vi "PSTR Offline Analysis.vi"() -> ()   [LabVIEW 2020]
uses:
  <vilib>/printing/EasyPrintingControls.llb/layout_options.ctl
  <vilib>/printing/EasyPrintingControls.llb/orientation.ctl
  <vilib>/printing/EasyPrintingControls.llb/panel_scaling_for_page.ctl
  <vilib>/printing/EasyPrintingControls.llb/margins.ctl
  <vilib>/printing/EasyPrintingControls.llb/margin_values.ctl
  <vilib>/printing/EasyPrintingControls.llb/measurement_system.ctl
  <vilib>/printing/EasyPrintingControls.llb/printer_options.ctl
  <vilib>/printing/EasyPrintingControls.llb/printing_method.ctl
  <vilib>/printing/EasyPrintingControls.llb/color_or_monochrome.ctl
  <vilib>/printing/EasyPrintingControls.llb/page_header_options.ctl
  <vilib>/printing/EasyPrintingControls.llb/page_headers.ctl
  <vilib>/printing/EasyPrintingControls.llb/page_header_content_options.ctl
  PSTR VIs/Typedefs/PSTR-Data.ctl
  PSTR VIs/Typedefs/PSTR-Model Fit.ctl
  PSTR VIs/Typedefs/PSTR-Fit Parameters.ctl
  Utility VIs/Buttons/KCheckmarkBoolean 2.ctl
  PSTR VIs/Typedefs/PSTR-File Info.ctl
  PSTR VIs/Typedefs/PSTR-Parameters.ctl
  PSTR VIs/Typedefs/PSTR-Stimulus Params.ctl
  Utility VIs/Type Defs/Left-Right ring.ctl
  PSTR VIs/Typedefs/PSTR-FreqSeq Params.ctl
  PSTR VIs/Typedefs/PSTR-LevelSeq Params.ctl
  PSTR VIs/Typedefs/PSTR-SeqParams.ctl
  PSTR VIs/Typedefs/PSTR-Response Params.ctl
  PSTR VIs/Typedefs/PSTR-Hidden Params.ctl
  PSTR VIs/Typedefs/PSTR-Window Shape.ctl
  Typedefs/PSTRA-Analysis State.ctl
  <vilib>/printing/EasyPrintingControls.llb/contents.ctl
  <vilib>/printing/EasyPrinting.llb/Easy Print VI Panel or Documentation (refnum).vi
  <vilib>/Utility/NIReport.llb/NI_ReportGenerationCore.lvlib
panel:
  out "CFTS-PSTR":T1
  in  "Mat Button":bool
  out "progress":dbl(slide) caption="2 kHz" scale=0.0..1.0
  in  "Reanalyze Button":bool
  out "Info":string
  in  "Path":path
  in  "Response":T2={"Grass gain"=10000.0, "Window (ms)"=10000.0, "Window shape"=enum."NONE", "NFFT"=10000}
  in  "Cancel Button":bool
  in  "Tabs":enum32{"Gain", "PSTR"}(tab)
  out "Spectrum":cluster{dbl, "dx":dbl, "Y":dbl[]}[](graph)
  out "vsFreq":cluster{"Array":dbl[], "Array":dbl[]}[](graph)
  in  "Legend":i32(listbox)
  out "Gain":cluster{"Array":dbl[], "Array":dbl[]}[](graph)
  in  "iFreq":u16(ring) items=["2 kHz"]
  out "RespAmp":cluster{"Array":dbl[], "Array":dbl[]}[](graph)
  in  "Show fits":T3
  in  "iFreq 2":u16(ring) items=["2 kHz"]
  in  "Legend 2":i32(listbox)
  in  "Separation (uV)":dbl min=0.0 step=1.0
  out "FitSummary":cluster{"Array":dbl[], "Array":dbl[]}[](graph)
  out "PSTH":cluster{"Array":dbl[], "Array":dbl[]}[](graph)
  out "finished":errorcluster
  out "Result":cluster{"Data":T4, "error":errorcluster}
  in  "layout options":T7={"orientation (unchanged)"=0, "panel scaling for page (unchanged)"=0, "margins"={"override VI margins (false)"=FALSE, "margins (1.00)"={"top"=1.0, "left"=1.0, "right"=1.0, "bottom"=1.0}, "measurement system (default)"=0}, "printer options"={"destination printer name (current)"="", "printing method (unchanged)"=0, "color or monochrome (unchanged)"=0}, "page header options"={"page headers (unchanged)"=0, "page header content options"={"Include VI Name"=TRUE, "Include VI Path"=TRUE, "Include Last Modification Date"=TRUE, "Include Date Printed"=TRUE, "Include Page Number"=TRUE, "Include VI Icon"=TRUE}}} {"page header options"."page headers (unchanged)" items=["Unchanged", "Include page headers", "Do not include page headers"]; "printer options"."color or monochrome (unchanged)" items=["Unchanged", "Color/grayscale", "Monochrome"]; "printer options"."printing method (unchanged)" items=["Unchanged", "Standard", "PostScript", "Bitmap"]; "panel scaling for page (unchanged)" items=["Unchanged", "No Scaling", "Scale front panel to fit"]; "orientation (unchanged)" items=["Unchanged", "portrait", "landscape"]; "margins"."measurement system (default)" items=["Default", "US", "Metric"]; "margins"."margins (1.00)"."right" format="%.2f"; "margins"."margins (1.00)"."bottom" format="%.2f"; "margins"."margins (1.00)"."top" format="%.2f"; "margins"."margins (1.00)"."left" format="%.2f"}
  # "PSTR Analysis"
  # "NF x NL x 2 x Npts"
  # "NF x NL x Npts"
  # "NF x NL"
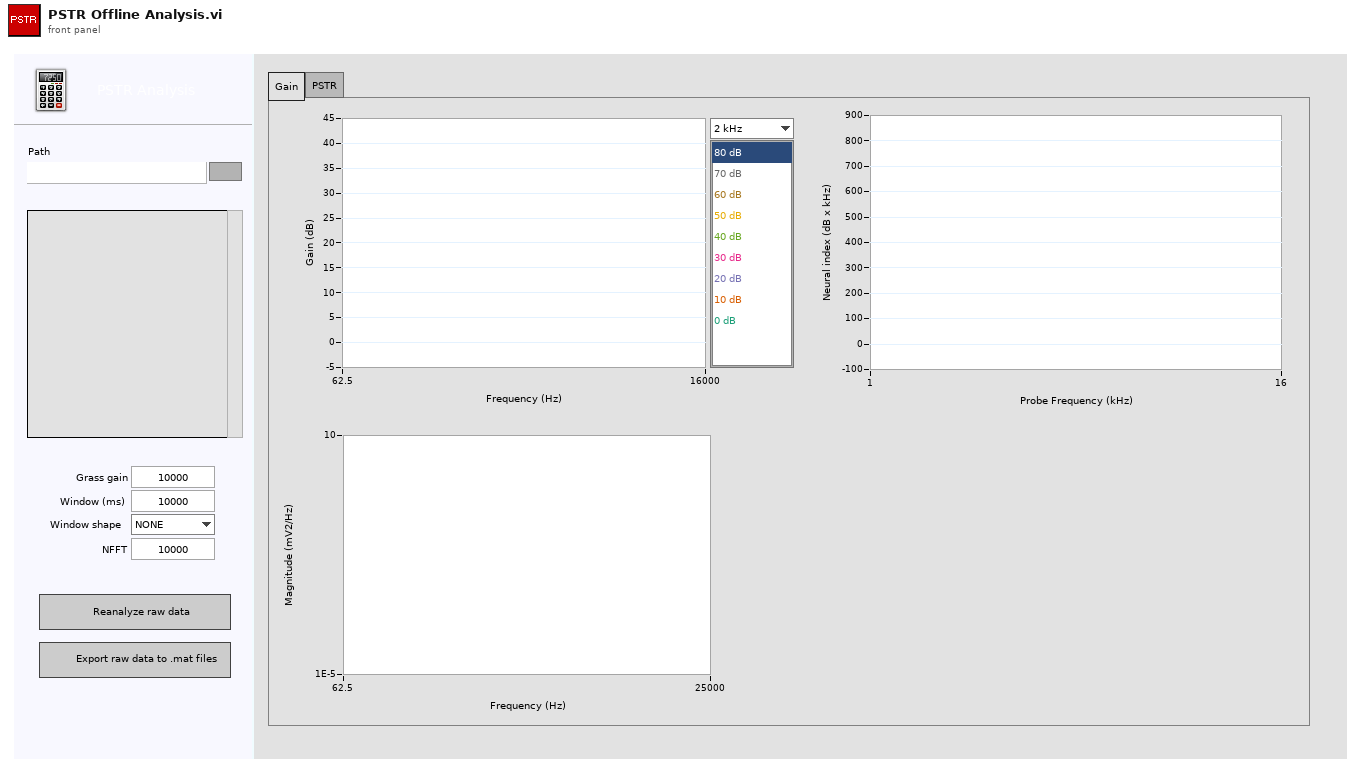
[diagram p1: front panel]
types:
  T1 = typedef "PSTR-File Info.ctl" = cluster{"Date":string, "Filename":string, "Version":i32, "Notes":string}
  T2 = cluster{"Grass gain":dbl, "Window (ms)":dbl, "Window shape":enum16{"NONE", "Hamming"}, "NFFT":i32}
  T3 = typedef "KCheckmarkBoolean 2.ctl" = bool
  T4 = typedef "PSTR-Data.ctl" = cluster{"Freq":dbl[], "Level":dbl[], "order":i32[], "PSD":dbl[][][][], "Gain":dbl[][][], "Index":dbl[][], "iFreq":i32, "df":dbl, "User":string, "ID":i32, "Run":i32, "iLevel":i32, "finished":bool, "resumed":bool, "Spont":dbl[][], "PSTR":dbl[][][], "dt":dbl, "delay":dbl, "durat":dbl, "Fits":T5[][], "Amplitude":dbl[][]}
  T5 = typedef "PSTR-Model Fit.ctl" = cluster{"Parameters":T6, "t":dbl[], "y":dbl[], "R2":dbl}
  T6 = typedef "PSTR-Fit Parameters.ctl" = cluster{"Ar":dbl, "Tr":dbl, "Ast":dbl, "Tst":dbl, "Ass":dbl}
  T7 = typedef "NI_ReportGenerationCore.lvlib/layout_options.ctl" = cluster{"orientation (unchanged)":T8, "panel scaling for page (unchanged)":T9, "margins":T10, "printer options":T13, "page header options":T16}
  T8 = typedef "NI_ReportGenerationCore.lvlib/orientation.ctl" = u16
  T9 = typedef "NI_ReportGenerationCore.lvlib/panel_scaling_for_page.ctl" = u16
  T10 = typedef "NI_ReportGenerationCore.lvlib/margins.ctl" = cluster{"override VI margins (false)":bool, "margins (1.00)":T11, "measurement system (default)":T12}
  T11 = typedef "NI_ReportGenerationCore.lvlib/margin_values.ctl" = cluster{"top":dbl, "left":dbl, "right":dbl, "bottom":dbl}
  T12 = typedef "NI_ReportGenerationCore.lvlib/measurement_system.ctl" = u16
  T13 = typedef "NI_ReportGenerationCore.lvlib/printer_options.ctl" = cluster{"destination printer name (current)":string, "printing method (unchanged)":T14, "color or monochrome (unchanged)":T15}
  T14 = typedef "NI_ReportGenerationCore.lvlib/printing_method.ctl" = u16
  T15 = typedef "NI_ReportGenerationCore.lvlib/color_or_monochrome.ctl" = u16
  T16 = typedef "NI_ReportGenerationCore.lvlib/page_header_options.ctl" = cluster{"page headers (unchanged)":T17, "page header content options":T18}
  T17 = typedef "NI_ReportGenerationCore.lvlib/page_headers.ctl" = u16
  T18 = typedef "NI_ReportGenerationCore.lvlib/page_header_content_options.ctl" = cluster{"Include VI Name":bool, "Include VI Path":bool, "Include Last Modification Date":bool, "Include Date Printed":bool, "Include Page Number":bool, "Include VI Icon":bool}
  T19 = typedef "PSTRA-Analysis State.ctl" = cluster{"Last folder":path, "separation":dbl}
  T20 = typedef "PSTR-Parameters.ctl" = cluster{"Stimulus":T21, "FreqSeq":T23, "LevelSeq":T24, "Seq":T25, "Response":T26, "Hidden":T27, "RejThr":dbl}
  T21 = typedef "PSTR-Stimulus Params.ctl" = cluster{"Ear":T22, "BW (oct)":dbl, "Seed":i32, "Ramp (ms)":dbl, "On time (ms)":dbl, "Off time (ms)":dbl, "Delay (ms)":dbl}
  T22 = typedef "Left-Right ring.ctl" = enum16{"Right", "Left"}
  T23 = typedef "PSTR-FreqSeq Params.ctl" = cluster{"Min (kHz)":dbl, "Max (kHz)":dbl, "Step (oct)":dbl}
  T24 = typedef "PSTR-LevelSeq Params.ctl" = cluster{"Min (dB)":dbl, "Max (dB)":dbl, "Step (dB)":dbl}
  T25 = typedef "PSTR-SeqParams.ctl" = cluster{"Order":enum16{"Sequential", "Random"}, "Averages":i32}
  T26 = typedef "PSTR-Response Params.ctl" = cluster{"Grass gain":dbl, "Window (ms)":dbl}
  T27 = typedef "PSTR-Hidden Params.ctl" = cluster{"Sample rate (Hz)":dbl, "Nfft":i32, "save raw":bool, "sep":dbl, "Window":T28}
  T28 = typedef "PSTR-Window Shape.ctl" = enum16{"NONE", "Hamming"}
  T29 = cluster{enum16{"Reprocess", "Export"}, path, "PSTR Params":T20}
  T30 = typedef "PSTR-SCL Element.ctl" = cluster{"raw file":path, "iFreq":i32, "iLevel":i32, "spont":bool}
  T31 = typedef "PSTR-Runtime Data.ctl" = cluster{"Fs":dbl, "AOpts":i32, "stimChan":T32, "len":i32, "offset1":i32, "iLevel":i32, "AOChan":i32[], "Level":dbl[], "nacc":i32, "nrej":i32, "nacq":i32, "abort":bool, "offset2":i32, "gain":dbl, "Nfft":i32, "Neural":dbl[], "Micro":dbl[], "raw":refnum<file>, "spont":bool, "PSTR":dbl[], "trialLen":i32, "gate":dbl[], "window":u16, "BP":cluster{"reverse":dbl[], "forward":dbl[]}, "Smooth":cluster{"reverse":dbl[], "forward":dbl[]}}
  T32 = typedef "Stimulus Channel (Full).xctl/Full Stimulus Channel Data.ctl" = cluster{"Waveform":T33, "Filter":T50, "Burst":T52, "Level":T53, "Name":string, "Advanced":T55, "SAM":T56}
  T33 = typedef "Waveform XCtl.xctl/Waveform Data.ctl" = cluster{"Type":T34, "Tone":T35, "Pulse Train":T36, "Noise":T39, "File":T40, "FMSweep":T41, "Chirp Train":T42, "Complex Tone":cluster{"Params":T44, "Data":T46}, "Moving Ripple":T47}
  T34 = typedef "Waveform Enum.ctl" = enum16{"OFF", "Tone", "Noise", "Pulse Train", "File", "FM Sweep", "Chirp Train", "Complex Tone", "FM Tone", "Moving Ripple"}
  T35 = typedef "Tone Params.ctl" = cluster{"Frequency (kHz)":dbl, "Last Freq":dbl, "Last Phase":dbl}
  T36 = typedef "Pulse Train Params.ctl" = cluster{"Pulse width (us)":dbl, "Pulse rate (Hz)":dbl, "Gap (ms)":dbl, "Polarity":T37, "PT State":T38, "Asynch":bool}
  T37 = typedef "Pulse Polarity.ctl" = enum16{"POS", "NEG", "POS-NEG", "NEG-POS"}
  T38 = typedef "PT-Continuous State.ctl" = cluster{"Template":dbl[], "Nperiod":i32, "Index":i32, "Pulse Rate (Hz)":dbl, "Phase (cycles)":dbl, "Noff":i32}
  T39 = typedef "Noise Params.ctl" = cluster{"InvFilt":bool, "Noise":dbl[], "CurPt":i32, "Aweight":bool, "Seed":i32, "afile":path}
  T40 = typedef "StimFile-Params.ctl" = cluster{"Filename":path, "Signal":dbl[], "Channel":i32, "stream":bool, "offset":i32, "nreps":i32, "loops":i32, "Randomize":bool, "order":i32[], "Seed":i32, "Tokens":i32}
  T41 = typedef "FM Sweep Params.ctl" = cluster{"Rate (oct/s)":dbl, "Fmin (Hz)":dbl, "Fmax (Hz)":dbl, "Ramp (ms)":dbl, "Linear":bool}
  T42 = typedef "Chirp Train.ctl" = cluster{"Params":T43, "Data":cluster{"WF":dbl[]}}
  T43 = typedef "Chirp Train Params.ctl" = cluster{"Fmin (kHz)":dbl, "Fmax (kHz)":dbl, "Compensate":bool, "Duration (ms)":dbl}
  T44 = typedef "CT-Params.ctl" = cluster{"F0 (Hz)":dbl, "Band":cluster{"Flow (Hz)":dbl, "Fhigh (Hz)":dbl}, "Phase":T45, "Min F0 (Hz)":dbl, "Max F0 (Hz)":dbl, "ContinRandPhase":bool, "Max peak factor":dbl, "Max mod depth":dbl, "MinHarmNum":i32, "MaxHarmNum":i32, "Level Mode":enum16{"per component", "overall rms"}, "% jitter":dbl}
  T45 = typedef "CT-Phase Enum.ctl" = enum16{"Cosine", "Random", "Alternating"}
  T46 = typedef "CT-Runtime Data.ctl" = cluster{"Ncomp":i32, "MinHarm":i32, "Phase":dbl[], "Amplitude":dbl[], "Npts/frame":i32, "Last F0":dbl, "Fmin":dbl, "Fmax":dbl, "Lslope":dbl, "randphase":bool, "overall rms":bool, "fmult":dbl[], "jittered":bool}
  T47 = typedef "Moving Ripple.ctl" = cluster{"Params":T48, "Data":T49}
  T48 = typedef "Moving Ripple.Params.ctl" = cluster{"Fmin":dbl, "Fmax":dbl, "Density":dbl, "Velocity":dbl, "Depth":dbl, "Phase":dbl, "Comp/oct":i32}
  T49 = typedef "Moving Ripple.Data.ctl" = cluster{"Freq":dbl[], "A":dbl[], "phase":dbl[], "Phase":dbl}
  T50 = typedef "Advanced Filter XCtl.xctl/Filter Data.ctl" = cluster{"Type":enum16{"Lowpass", "Highpass", "Bandpass", "Bandstop", "OFF"}, "CF (kHz)":dbl, "BW (kHz)":dbl, "Cascade":bool, "Quadrature":bool, "Scale Factor":dbl, "Stages":cluster{"IIR Filter":cluster{"filter structure":enum32{"IIR 2nd Order", "IIR 4th Order"}, "Reverse Coefficients":dbl[], "Forward Coefficients":dbl[]}, "State":dbl[]}[], "Class":enum16{"Elliptic", "Butterworth"}, "Order":i32, "BWUnits":T51}
  T51 = typedef "Filter-Bandwidth Units.ctl" = enum16{"Linear", "Octaves", "Min-Max"}
  T52 = typedef "Burst Control.xctl/Burst Data.ctl" = cluster{"Active":bool, "Delay (ms)":dbl, "Duration (ms)":dbl, "Ramp (ms)":dbl, "Rate (Hz)":dbl, "Trepeat (ms)":dbl, "Repeat":bool}
  T53 = typedef "Level XCtl.xctl/Level Data.ctl" = cluster{"Level":dbl, "Units":T54, "Max":dbl, "Multiplier":dbl, "Cal File":path, "Cal":cluster{"Freq (Hz)":dbl[], "Mag (dB SPL)":dbl[], "Phase (deg)":dbl[]}}
  T54 = typedef "Level Units.ctl" = enum16{"dB atten", "dB SPL", "dB re 1 Vrms", "dB V/Hz½", "mW", "dB HL", "Volts", "dB mW"}
  T55 = typedef "Advanced Stimulus Options.xctl/Advanced Stimulus Options.ctl" = cluster{"Rep Mask":string, "AltPol":bool, "Var":string, "Expr":string, "Persist":bool}
  T56 = typedef "SAM Params.ctl" = cluster{"Active":bool, "Frequency (Hz)":dbl, "Depth":dbl, "Init Phase (cycles)":dbl, "phase (degrees)":dbl, "Asynch":bool}
  T57 = enum8{"Enabled", "Disabled", "Disabled and Grayed Out"}
  T58 = typedef "NI_ReportGenerationCore.lvlib/contents.ctl" = u16
  T59 = cluster{enum16{"Reprocess", "Export"}, "Path":path, "PSTR Params":T20}
  T60 = cluster{"Grass gain":dbl, "Window (ms)":dbl, "Window":T28, "Nfft":i32}
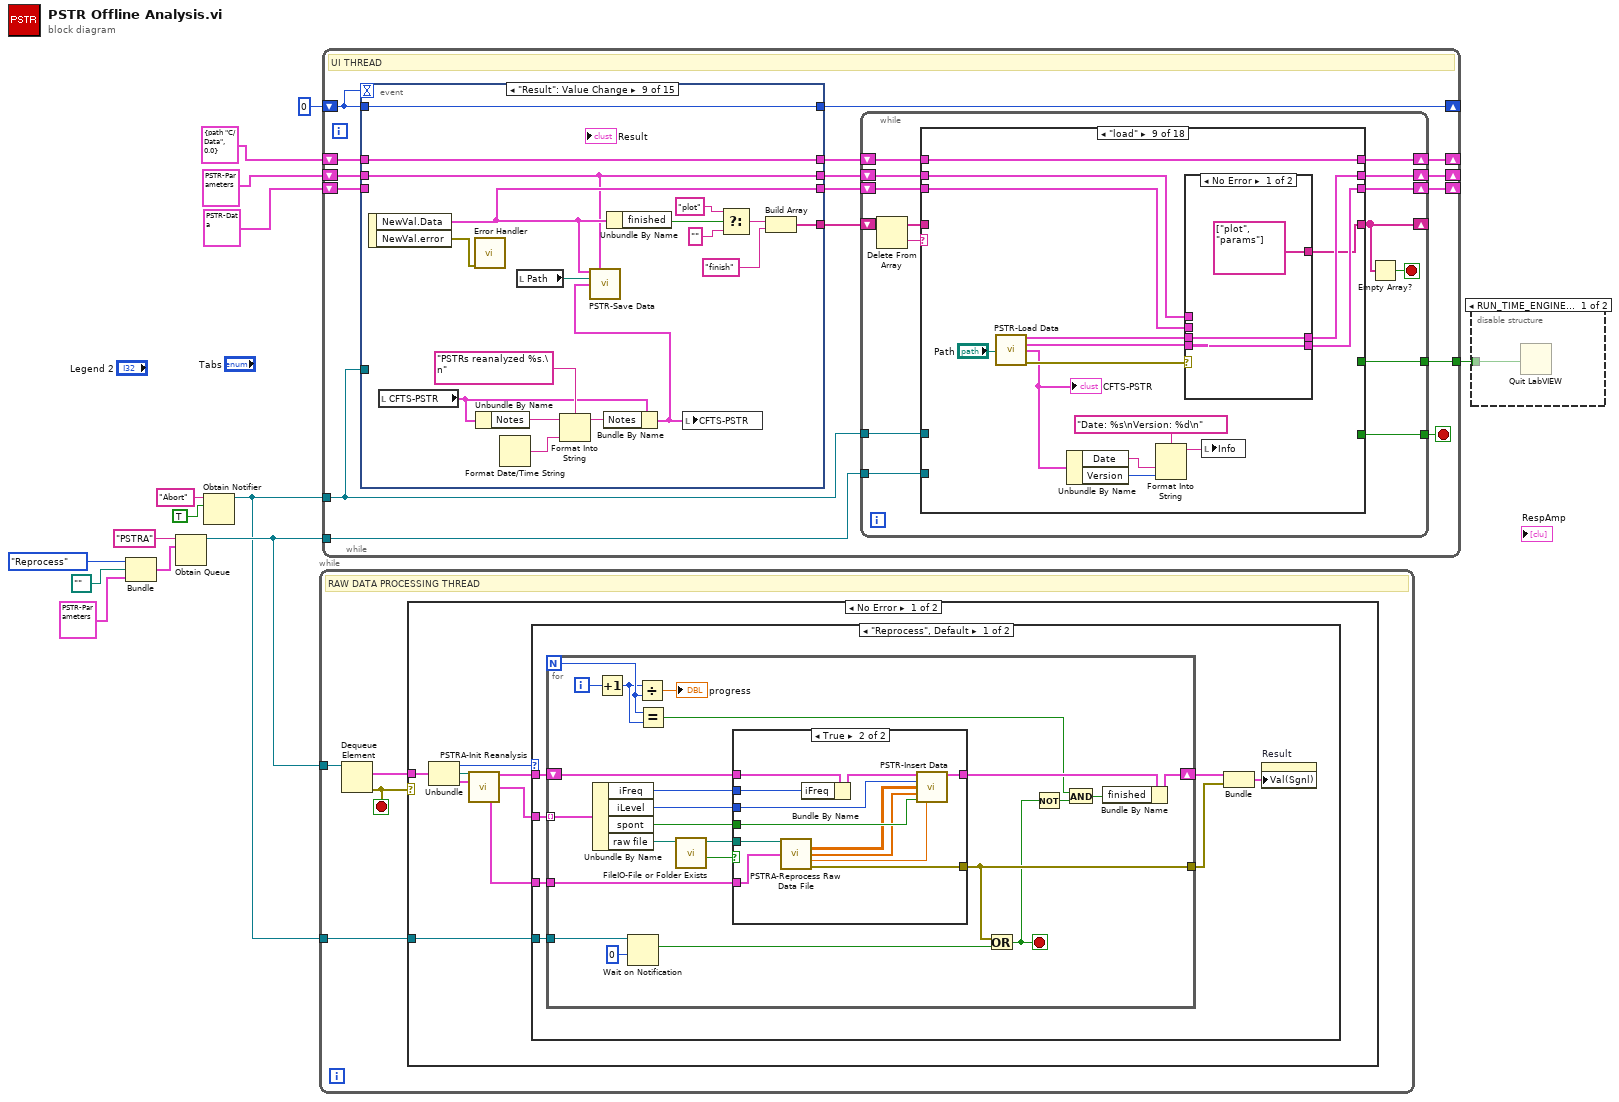
[diagram p0: block diagram]
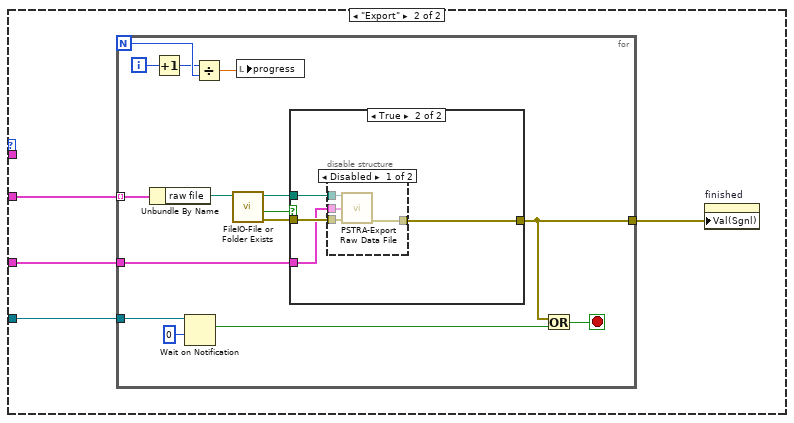
[diagram p4: hidden frame]
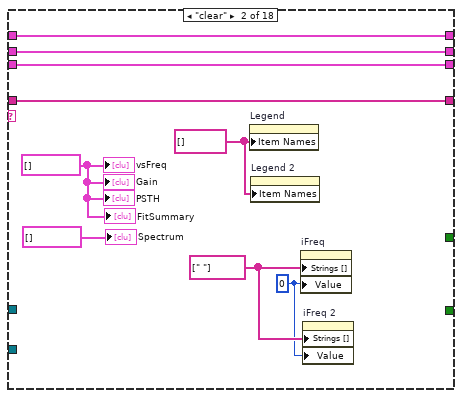
[diagram p9: hidden frame]
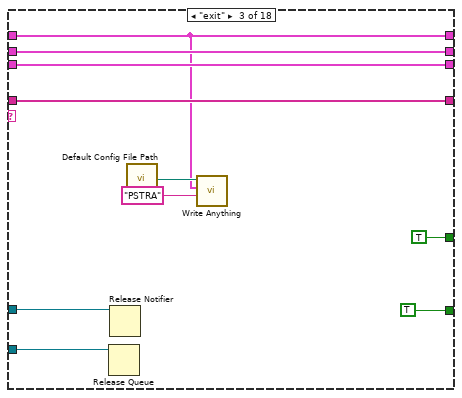
[diagram p10: hidden frame]
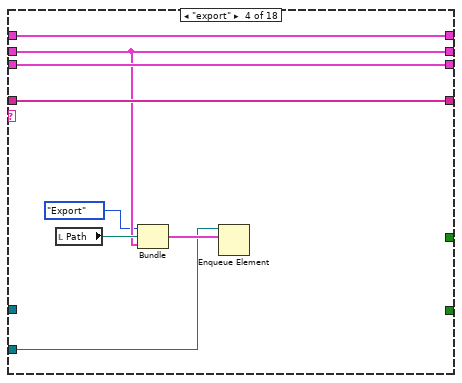
[diagram p11: hidden frame]
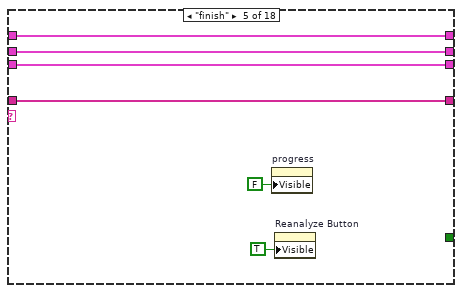
[diagram p12: hidden frame]
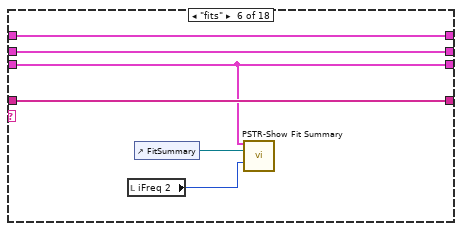
[diagram p13: hidden frame]
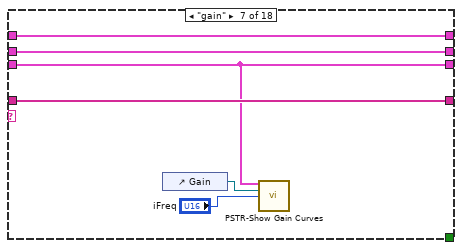
[diagram p14: hidden frame]
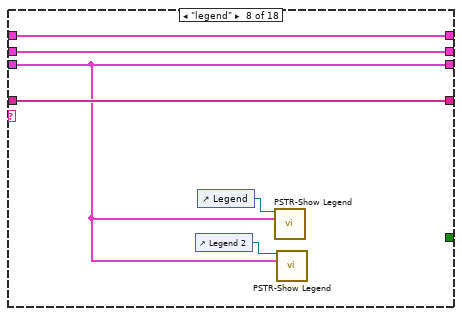
[diagram p15: hidden frame]
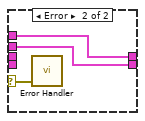
[diagram p16: hidden frame]
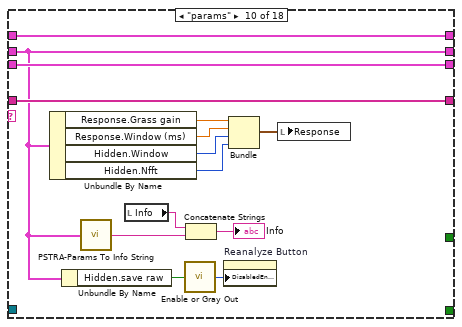
[diagram p17: hidden frame]
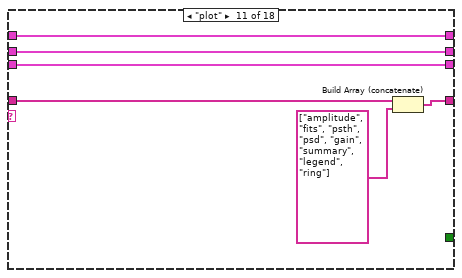
[diagram p18: hidden frame]
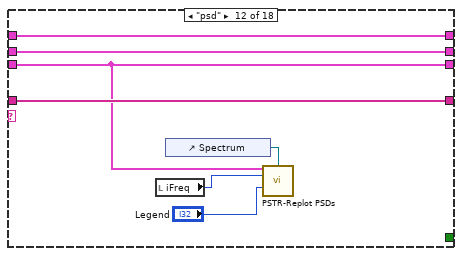
[diagram p19: hidden frame]
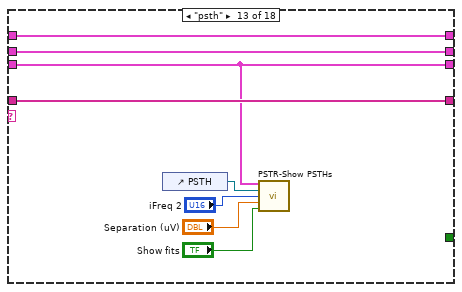
[diagram p20: hidden frame]
diagram:
  n1 = Bundle(enum16{"Reprocess", "Export"}."Reprocess", path "", "PSTR Params"=T20 {"Stimulus"={"Ear"=enum."Right", "BW (oct)"=673.0, "Seed"=6, "Ramp (ms)"=10000.0, "On time (ms)"=10000.0, "Off time (ms)"=10000.0, "Delay (ms)"=10000.0}, "FreqSeq"={"Min (kHz)"=10000.0, "Max (kHz)"=10000.0, "Step (oct)"=10000.0}, "LevelSeq"={"Min (dB)"=10000.0, "Max (dB)"=10000.0, "Step (dB)"=10000.0}, "Seq"={"Order"=enum."Sequential", "Averages"=6}, "Response"={"Grass gain"=10000.0, "Window (ms)"=0.0}, "Hidden"={"Sample rate (Hz)"=20000.0, "Nfft"=0, "save raw"=FALSE, "sep"=0.0, "Window"=enum."NONE"}, "RejThr"=0.0}) -> (w10:T29)  [unwired: 1 in]
  n2 = Obtain Queue(name (unnamed)="PSTRA", element data type=w10) -> (queue out=w14:refnum<queue>)  [unwired: 3 in, 2 out]
  n3 = Obtain Notifier(name (unnamed)="Abort", notification data type=TRUE) -> (notifier out=w5:refnum<notifier>)  [unwired: 2 in, 2 out]
  n4 = while {
    tunnel: w14 -> [w18]
    tunnel: w5 -> [w15]
    stop <- w17 stop-if-true
    # "RAW DATA PROCESSING THREAD"
    n5 = Dequeue Element(queue=w18) -> (element=w16:T29, error out=w17:errorcluster)  [unwired: 2 in, 2 out]
    n6 = case shown="No Error" w17 {
      tunnel: w16 -> [w26 _]
      tunnel: w15 -> [w23 _]
      frame No Error {
        n7 = Unbundle(w26) -> (w19:enum16{"Reprocess", "Export"}, w21:path, "PSTR Params"=w20:T20)
        n8 = call "PSTRA-Init Reanalysis.vi"("Path"=w21, "PSTR Params"=w20) -> ("Data"=w25:T4, "SCL"=w24:T30[], "Runtime out"=w22:T31)  [unwired: 11 in]
        n9 = case shown="\"Reprocess\", Default" w19 {
          tunnel: w25 -> [w33 _]
          tunnel: w24 -> [w32 w73]
          tunnel: w23 -> [w29 w72]
          tunnel: w22 -> [w27 w70]
          frame "Reprocess", Default {
            n10 = for {
              N -> [w45]
              tunnel: w32 -> [w47] mode=indexing
              shift-right: [w43] -> w31
              shift-left: w33 -> [w50]
              tunnel: w29 -> [w53]
              tunnel: [w40] -> w28
              tunnel: w27 -> [w37]
              i -> [w56]
              stop <- w39 stop-if-true
              n11 = Unbundle By Name(w47) -> ("iFreq"=w35:i32, "iLevel"=w34:i32, "spont"=w36:bool, "raw file"=w51:path)
              n12 = Increment(x=w56) -> (x+1=w44:i32)
              n13 = Wait on Notification(notifier=w53, timeout in ms (-1)=0) -> (notification=w52:bool)  [unwired: 2 in, 3 out]
              n14 = Divide(x=w44, y=w45) -> (x/y=→"progress":dbl)
              n15 = Equal?(x=w45, y=w44) -> (x = y?=w42:bool)
              n16 = call "FileIO-File or Folder Exists.vi"("path"=w51) -> ("Exists?"=w48:bool, "dup path"=w46:path)  [unwired: 7 in, 2 out]
              n17 = case shown="True" w48 {
                tunnel: w50 -> [w57 w69]
                tunnel: [w57 w68] -> w49
                tunnel: w46 -> [_ w66]
                tunnel: [_ w67] -> w40
                tunnel: w37 -> [_ w65]
                tunnel: w36 -> [_ w61]
                tunnel: w35 -> [_ w63]
                tunnel: w34 -> [_ w62]
                frame False {
                }
                frame True {
                  n18 = call "PSTRA-Reprocess Raw Data File.vi"("Path"=w66, "Runtime in"=w65) -> ("PSD"=w60:dbl[][], "PSTH"=w59:dbl[], "Amplitude"=w58:dbl, "error out"=w67:errorcluster)  [unwired: 9 in, 1 out]
                  n19 = Bundle By Name(cluster=w69, "iFreq"=w63) -> (w64:T4)
                  n20 = call "PSTR-Insert Data.vi"("Data in"=w64, "iLevel"=w62, "PSD"=w60, "PSTR"=w59, "Spont"=w61, "Amplitude"=w58) -> ("Data out"=w68:T4)  [unwired: 9 in]
                }
              }
              n21 = Or(x=w40, y=w52) -> (x .or. y?=w39:bool)
              n22 = Not(x=w39) -> (.not. x?=w41:bool)
              n23 = And(x=w42, y=w41) -> (x .and. y?=w38:bool)
              n24 = Bundle By Name(cluster=w49, "finished"=w38) -> (w43:T4)
            }
            n25 = Bundle("Data"=w31, "error out"=w28) -> (w30:cluster{"Data":T4, "error out":errorcluster})  [unwired: 1 in]
            n26 = property on="Result" class="Clust (strict)"("Val(Sgnl)"=w30) -> ()  [unwired: 2 in, 2 out]
          }
          frame "Export" {
            n27 = for {
              N -> [w80]
              tunnel: w73 -> [w82] mode=indexing
              tunnel: w72 -> [w86]
              tunnel: [w78] -> w71
              tunnel: w70 -> [w74]
              i -> [w88]
              stop <- w77 stop-if-true
              n28 = Unbundle By Name(w82) -> ("raw file"=w84:path)
              n29 = Increment(x=w88) -> (x+1=w79:i32)
              n30 = Wait on Notification(notifier=w86, timeout in ms (-1)=0) -> (notification=w85:bool)  [unwired: 2 in, 3 out]
              n31 = Divide(x=w79, y=w80) -> (x/y=w76:dbl)
              n32 = call "FileIO-File or Folder Exists.vi"("path"=w84) -> ("error out"=w75:errorcluster, "Exists?"=w83:bool, "dup path"=w81:path)  [unwired: 7 in, 1 out]
              n33 = local write "progress"(w76) -> ()
              n34 = case shown="True" w83 {
                tunnel: w81 -> [_ w92]
                tunnel: [_ w90] -> w78
                tunnel: w75 -> [_ w91]
                tunnel: w74 -> [_ w89]
                frame False {
                }
                frame True {
                  n35 = disable-structure shown="Disabled" {
                    disable-tunnel: w92 -> [w96 _]
                    disable-tunnel: w91 -> [w95 _]
                    disable-tunnel: [w94 _] -> w90
                    disable-tunnel: w89 -> [w93 _]
                    frame Disabled {
                      n36 = call "PSTRA-Export Raw Data File.vi"("Path"=w96, "Runtime in"=w93, "error in (no error)"=w95) -> ("error out"=w94:errorcluster)  [unwired: 12 in]
                    }
                    frame Enabled {
                    }
                  }
                }
              }
              n37 = Or(x=w78, y=w85) -> (x .or. y?=w77:bool)
            }
            n38 = property on="finished" class="Clust (strict)"("Val(Sgnl)"=w71) -> ()  [unwired: 2 in, 2 out]
          }
        }
      }
      frame Error {
      }
    }
  }
  n39 = while {
    tunnel: w14 -> [w101]
    shift-right: [w112] -> _
    shift-left: 0 -> [w110]
    shift-right: [w107] -> _
    shift-left: T20 {"Stimulus"={"Ear"=enum."Right", "BW (oct)"=0.3333, "Seed"=37, "Ramp (ms)"=5.0, "On time (ms)"=300.0, "Off time (ms)"=300.0, "Delay (ms)"=10000.0}, "FreqSeq"={"Min (kHz)"=4.0, "Max (kHz)"=64.0, "Step (oct)"=0.5}, "LevelSeq"={"Min (dB)"=0.0, "Max (dB)"=80.0, "Step (dB)"=20.0}, "Seq"={"Order"=enum."Sequential", "Averages"=100}, "Response"={"Grass gain"=10000.0, "Window (ms)"=200.0}, "Hidden"={"Sample rate (Hz)"=100000.0, "Nfft"=2048, "save raw"=FALSE, "sep"=0.0, "Window"=enum."NONE"}, "RejThr"=15.0} ("PSTR Params") -> [w111]
    shift-right: [w103] -> _
    shift-left: T4 {"Freq"=[], "Level"=[], "order"=[], "PSD"=[], "Gain"=[], "Index"=[], "iFreq"=0, "df"=0.0, "User"="", "ID"=0, "Run"=0, "iLevel"=0, "finished"=FALSE, "resumed"=FALSE, "Spont"=[], "PSTR"=[], "dt"=0.0, "delay"=0.0, "durat"=0.0, "Fits"=[], "Amplitude"=[]} ("Data") -> [w105]
    tunnel: w5 -> [w102]
    shift-right: [w98] -> _
    shift-left: T19 {"Last folder"=path "C:/Data", "separation"=0.0} ("Cluster") -> [w100]
    tunnel: [w97] -> w1
    stop <- w106 stop-if-true
    # "UI THREAD"
    n40 = event shown="[8] \"Result\": Value Change" {
      selector: _ -> [_ _ _ _ _ _ _ _ _ _ _ _ _ _ _]
      dyn-events: _ -> [_ _ _ _ _ _ _ _ _ _ _ _ _ _ _]
      timeout: w110 -> [_ _ w327 _ _ _ _ _ _ _ _ _ _ _ _]
      tunnel: [-1 w314 w327 w335 w345 w354 w361 w368 w386 w392 w399 w404 w409 w416 w421] -> w112
      tunnel: w111 -> [w308 w311 w325 w334 w344 w353 w360 w367 w376 w391 w398 w403 w408 w415 w420]
      tunnel: [w308 w311 w325 w334 w341 w353 w360 w367 w376 w391 w398 w403 w408 w415 w420] -> w108
      tunnel: w110 -> [_ w314 _ w335 w345 w354 w361 w368 w386 w392 w399 w404 w409 w416 w421]
      tunnel: [string[] ["restore", "clear"] w313 string[] ["exit"] ("f") string[] ["load"] ("f") _ string[] ["reanalyze", "clear"] ("f") string[] ["export"] ("f") _ w383 string[] ["finish"] ("f") string[] ["psd", "gain"] ("f") string[] ["fits", "psth"] ("f") string[] ["psd"] ("f") string[] ["psth"] ("f") string[] ["psth"] ("f")] -> w109
      tunnel: w105 -> [w307 w312 w323 w333 w343 w352 w359 w366 _ w390 w397 w402 w407 w414 w419]
      tunnel: [w307 w312 w323 w333 w343 w352 w359 w366 w377 w390 w394 w402 w407 w414 w419] -> w104
      tunnel: w102 -> [_ _ _ _ _ _ _ w362 _ _ _ _ _ _ _]
      tunnel: w100 -> [w303 w310 w322 w330 w342 w351 w358 w365 w385 w389 w395 w400 w406 w413 w418]
      tunnel: [w303 w310 w322 w329 w342 w351 w358 w365 w385 w389 w395 w400 w406 w412 w418] -> w99
      event Timeout {
        n41 = event-data() -> ()  [unwired: 1 in, 1 out]
        n42 = property on="progress" class="Slide (strict)"("Visible"=FALSE) -> ()  [unwired: 2 in, 2 out]
        n43 = property on="Reanalyze Button" class="Bool"("DisabledEnum"=T57."Disabled and Grayed Out" ("Disabled"), "Visible"=TRUE) -> ()  [unwired: 2 in, 2 out]
        n44 = local write "Info"("" ("Info")) -> ()
        n45 = local write "Path"(path "" ("Path")) -> ()
      }
      event Menu Selection (User) {
        n46 = event-data() -> ("ItemTag"=w316:string)  [unwired: 1 in]
        n47 = case shown="\"mmFileExit\"" w316 {
          tunnel: [_ w317 _] -> w315
          tunnel: [_ _ string[] ["exit"]] -> w313
          frame "", Default {
          }
          frame "mmFilePrint" {
            w319 = T58 1 items=["Complete front panel", "Visible portion of front panel", "Icon, description, panel and diagram", "Documentation: Using the panel", "Documentation: Using as a subVI", "Documentation: Complete", "Documentation: Custom"] ("contents (complete front panel)")
            n48 = control-ref of="This VI"() -> (w318:refnum<vi>)
            n49 = call-poly <vilib>:"Easy Print VI Panel or Documentation.vi"("layout options"="layout options", "contents (complete front panel)"=w319, "VI reference"=w318) -> ("error out"=w317:errorcluster)  [unwired: 7 in, 1 out]
          }
          frame "mmFileExit" {
          }
        }
        n50 = call "Error Handler.vi"("error in (no error)"=w315) -> ()  [unwired: 13 in, 2 out]
      }
      event Panel Close? {
        n51 = event-data() -> ()  [unwired: 1 in, 1 out]
        n52 = event-data("Discard?"=TRUE) -> ()  [unwired: 1 in, 1 out]
      }
      event "Path": Value Change {
        n53 = event-data() -> ("NewVal"=w331:path)  [unwired: 1 in]
        n54 = Strip Path(path=w331) -> (stripped path=w328:path)  [unwired: 1 out]
        n55 = Bundle By Name(cluster=w330, "Last folder"=w328) -> (w329:T19)
        n56 = property on="Path" class="Path"("StartPath"=w328) -> ()  [unwired: 2 in, 2 out]
      }
      event "Response": Value Change {
        n57 = event-data() -> ()  [unwired: 1 in, 1 out]
        n58 = Unbundle By Name("Response") -> ("Grass gain"=w339:dbl, "Window (ms)"=w338:dbl, "NFFT"=w337:i32, "Window shape"=w336:enum16{"NONE", "Hamming"})
        n59 = Bundle By Name(cluster=w344, "Response.Grass gain"=w339, "Response.Window (ms)"=w338, "Hidden.Nfft"=w337, "Hidden.Window"=w336) -> (w341:T20)
      }
      event "Reanalyze Button": Value Change {
        n60 = event-data() -> ()  [unwired: 1 in, 1 out]
        n61 = property on="Reanalyze Button" class="Bool"("Visible"=FALSE) -> ()  [unwired: 2 in, 2 out]
        n62 = property on="Cancel Button" class="Bool"("DisabledEnum"=T57."Enabled" ("Disabled")) -> ()  [unwired: 2 in, 2 out]
        n63 = property on="progress" class="Slide (strict)"("Visible"=TRUE, "Value"=0.0 ("freq")) -> ()  [unwired: 2 in, 2 out]
      }
      event "Mat Button": Value Change {
        n64 = event-data() -> ()  [unwired: 1 in, 1 out]
        n65 = property on="progress" class="Slide (strict)"("Visible"=TRUE, "Value"=0.0 ("freq")) -> ()  [unwired: 2 in, 2 out]
      }
      event "Cancel Button": Value Change {
        n66 = event-data() -> ()  [unwired: 1 in, 1 out]
        n67 = Send Notification(notification=TRUE, notifier=w362) -> ()  [unwired: 1 in, 2 out]
        n68 = property on="Cancel Button" class="Bool"("DisabledEnum"=T57."Disabled and Grayed Out" ("Disabled")) -> ()  [unwired: 2 in, 2 out]
      }
      event "Result": Value Change {
        n69 = event-data() -> ("NewVal.Data"=w377:T4, "NewVal.error"=w384:errorcluster)  [unwired: 1 in]
        n70 = local read "CFTS-PSTR"() -> (w370:T1)
        n71 = call "Error Handler.vi"("error in (no error)"=w384) -> ()  [unwired: 13 in, 2 out]
        n72 = Unbundle By Name(w370) -> ("Notes"=w374:string)
        n73 = Format Date/Time String() -> (date/time string=w372:string)  [unwired: 3 in]
        n74 = local read "Path"() -> (w375:path)
        n75 = Format Into String(format string="PSTRs reanalyzed %s.\n", initial string=w374, w372) -> (resulting string=w371:string)  [unwired: 1 in, 1 out]
        n76 = Bundle By Name(cluster=w370, "Notes"=w371) -> (w369:T1)
        n77 = call "PSTR-Save Data.vi"("Data in"=w377, "PSTR Params"=w376, "path"=w375, "CFTS-PSTR"=w369) -> ()  [unwired: 9 in, 3 out]
        n78 = Unbundle By Name(w377) -> ("finished"=w381:bool)
        n79 = local write "CFTS-PSTR"(w369) -> ()
        n80 = Select(t="plot", s=w381, f="") -> (s? t:f=w379:string)
        n81 = Build Array(w379, "finish" ("String")) -> (w383:string[])
      }
      event "finished": Value Change {
        n82 = event-data() -> ("NewVal"=w388:errorcluster)  [unwired: 1 in]
        n83 = call "Error Handler.vi"("error in (no error)"=w388) -> ()  [unwired: 13 in, 2 out]
      }
      event "iFreq": Value Change {
        n84 = event-data() -> ("NewVal"=w393:u16)  [unwired: 1 in]
        n85 = Bundle By Name(cluster=w397, "iFreq"=w393) -> (w394:T4)
      }
      event "iFreq 2": Value Change {
        n86 = event-data() -> ()  [unwired: 1 in, 1 out]
      }
      event "Legend": Value Change {
        n87 = event-data() -> ()  [unwired: 1 in, 1 out]
      }
      event "Separation (uV)": Value Change {
        n88 = event-data() -> ("NewVal"=w411:dbl)  [unwired: 1 in]
        n89 = Bundle By Name(cluster=w413, "separation"=w411) -> (w412:T19)
      }
      event Value Change {
        n90 = event-data() -> ()  [unwired: 1 in, 1 out]
      }
    }
    n91 = while {
      shift-right: [w119] -> _
      shift-left: w109 -> [w127]
      shift-right: [w122] -> w107
      shift-left: w108 -> [w123]
      tunnel: w101 -> [w121]
      tunnel: [w120] -> w106
      shift-right: [w117] -> w103
      shift-left: w104 -> [w118]
      tunnel: w102 -> [w116]
      shift-right: [w114] -> w98
      shift-left: w99 -> [w115]
      tunnel: [w113] -> w97
      stop <- w125 stop-if-true
      n92 = Delete From Array(array=w127) -> (deleted portion=w126:string, array with subset deleted=w124:string[])  [unwired: 2 in]
      n93 = case shown="\"load\"" w126 {
        tunnel: w124 -> [w130 w139 w149 w158 w163 w169 w175 w182 _ w217 w222 w229 w237 w243 w252 w265 w287 w298]
        tunnel: w123 -> [w131 w140 w150 w154 w164 w170 w176 w181 w195 w207 w223 w230 w238 w244 w248 w256 w288 w299]
        tunnel: [w131 w140 w150 w154 w164 w170 w176 w181 w194 w207 w223 w230 w238 w244 w248 w256 w288 w299] -> w122
        tunnel: [w130 w139 w149 w158 w163 w169 w175 w182 w193 w217 w220 w229 w237 w243 w252 w265 w287 w298] -> w119
        tunnel: w121 -> [_ _ w148 w152 _ _ _ _ _ _ _ _ _ _ w246 _ _ _]
        tunnel: [_ _ TRUE _ _ _ _ _ _ _ _ _ _ _ _ _ _ _] -> w120
        tunnel: w118 -> [w129 w138 w146 w157 w162 w167 w172 w178 w197 w216 w218 w227 w235 w240 w251 w258 w282 w296]
        tunnel: [w129 w138 w146 w157 w162 w167 w172 w178 w196 w216 w218 w227 w235 w240 w251 w258 w282 w296] -> w117
        tunnel: w116 -> [_ _ w145 _ _ _ _ _ _ _ _ _ _ _ _ _ _ _]
        tunnel: w115 -> [w128 w137 w142 w156 w161 w166 w171 w179 w189 w215 w221 w226 w234 w242 w250 w257 w286 w295]
        tunnel: [w128 w137 w142 w156 w161 w166 w171 w179 w189 w215 w221 w226 w234 w242 w250 w255 w286 w295] -> w114
        tunnel: [_ _ TRUE _ _ _ _ _ _ _ _ _ _ _ _ _ _ _] -> w113
        frame "", Default {
        }
        frame "clear" {
          w134 = string[] [" "] ("Strings []")
          w133 = 0
          w135 = string[] [] ("Strings []")
          w132 = cluster{"Array":dbl[], "Array":dbl[]}[] [] ("vsFreq")
          n94 = property on="Legend" class="LstBox (strict)"("Item Names"=w135) -> ()  [unwired: 2 in, 2 out]
          n95 = property on="Legend 2" class="LstBox (strict)"("Item Names"=w135) -> ()  [unwired: 2 in, 2 out]
          n96 = property on="iFreq" class="Ring (strict)"("Strings []"=w134, "Value"=w133) -> ()  [unwired: 2 in, 2 out]
          n97 = property on="iFreq 2" class="Ring (strict)"("Strings []"=w134, "Value"=w133) -> ()  [unwired: 2 in, 2 out]
          "Spectrum" <- cluster{dbl, "dx":dbl, "Y":dbl[]}[] [] ("Spectrum")
          "vsFreq" <- w132
          "Gain" <- w132
          "PSTH" <- w132
          "FitSummary" <- w132
        }
        frame "exit" {
          n98 = Release Queue(queue=w148) -> ()  [unwired: 2 in, 3 out]
          n99 = Release Notifier(notifier=w145) -> ()  [unwired: 2 in, 3 out]
          n100 = call "Default Config File Path.vi"() -> ("Default config file name"=w144:path)
          n101 = call "Write Anything.vi"("Section Name (Name of \"Anything\")"="PSTRA" ("Section Name (Name of \"Type of Anything\")"), "Anything"=w142, "Path (dialog)"=w144) -> ()  [unwired: 7 in, 2 out]
        }
        frame "export" {
          n102 = local read "Path"() -> (w155:path)
          n103 = Bundle(enum16{"Reprocess", "Export"}."Export", "Path"=w155, "PSTR Params"=w154) -> (w153:T59)  [unwired: 1 in]
          n104 = Enqueue Element(queue=w152, element=w153) -> ()  [unwired: 2 in, 3 out]
        }
        frame "finish" {
          n105 = property on="progress" class="Slide (strict)"("Visible"=FALSE) -> ()  [unwired: 2 in, 2 out]
          n106 = property on="Reanalyze Button" class="Bool"("Visible"=TRUE) -> ()  [unwired: 2 in, 2 out]
        }
        frame "fits" {
          n107 = local read "iFreq 2"() -> (w165:u16)
          n108 = control-ref of="FitSummary"() -> (w168:refnum<vi>)
          n109 = call "PSTR-Show Fit Summary.vi"("Data"=w167, "XYGraph"=w168, "Freq index"=w165) -> ()  [unwired: 13 in]
        }
        frame "gain" {
          n110 = control-ref of="Gain"() -> (w174:refnum<vi>)
          n111 = call "PSTR-Show Gain Curves.vi"("Data"=w172, "XYGraph"=w174, "Freq"="iFreq") -> ()  [unwired: 13 in]
        }
        frame "legend" {
          n112 = control-ref of="Legend 2"() -> (w177:refnum<vi>)
          n113 = control-ref of="Legend"() -> (w180:refnum<vi>)
          n114 = call "PSTR-Show Legend.vi"("ListBox in"=w180, "Data"=w178) -> ()  [unwired: 14 in]
          n115 = call "PSTR-Show Legend.vi"("ListBox in"=w177, "Data"=w178) -> ()  [unwired: 14 in]
        }
        frame "load" {
          n116 = call "PSTR-Load Data.vi"("selected path"="Path") -> ("Params"=w191:T20, "Data"=w183:T4, "CFTS-PSTR"=w184:T1, "error out"=w192:errorcluster)  [unwired: 11 in]
          "CFTS-PSTR" <- w184
          n117 = Unbundle By Name(w184) -> ("Date"=w187:string, "Version"=w186:i32)
          n118 = Format Into String(format string="Date: %s\nVersion: %d\n", w187, w186) -> (resulting string=w185:string)  [unwired: 2 in, 1 out]
          n119 = case shown="No Error" w192 {
            selector: w192 -> [_ w203]
            tunnel: w195 -> [_ w202]
            tunnel: [w199 w202] -> w194
            tunnel: [w198 w201] -> w196
            tunnel: w197 -> [_ w201]
            tunnel: w191 -> [w199 _]
            tunnel: w183 -> [w198 _]
            tunnel: [string[] ["plot", "params"] _] -> w193
            frame No Error {
            }
            frame Error {
              n120 = call "Error Handler.vi"("error in (no error)"=w203) -> ()  [unwired: 13 in, 2 out]
            }
          }
          n121 = local write "Info"(w185) -> ()
        }
        frame "params" {
          n122 = Unbundle By Name(w207) -> ("Response.Grass gain"=w214:dbl, "Response.Window (ms)"=w213:dbl, "Hidden.Window"=w204:T28, "Hidden.Nfft"=w205:i32)
          n123 = Unbundle By Name(w207) -> ("Hidden.save raw"=w206:bool)
          n124 = call "PSTRA-Params To Info String.vi"("PSTR Params"=w207) -> ("Info"=w211:string)  [unwired: 14 in]
          n125 = local read "Info"() -> (w209:string)
          n126 = call "Enable or Gray Out.vi"("Boolean"=w206) -> ("Disabled"=w208:T57)
          n127 = Concatenate Strings(w209, w211) -> (→"Info":string)
          n128 = property on="Reanalyze Button" class="Bool"("DisabledEnum"=w208) -> ()  [unwired: 2 in, 2 out]
          n129 = Bundle("Grass gain"=w214, "Window (ms)"=w213, "Window"=w204, "Nfft"=w205) -> (w212:T60)  [unwired: 1 in]
          n130 = local write "Response"(w212) -> ()
        }
        frame "plot" {
          n131 = Build Array (concatenate)(w222, string[] ["amplitude", "fits", "psth", "psd", "gain", "summary", "legend", "ring"]) -> (w220:string[])
        }
        frame "psd" {
          n132 = local read "iFreq"() -> (w224:u16)
          n133 = control-ref of="Spectrum"() -> (w228:refnum<vi>)
          n134 = call "PSTR-Replot PSDs.vi"("Data"=w227, "Graph Ref"=w228, "ifreq"=w224, "ilevel"="Legend") -> ()  [unwired: 11 in, 1 out]
        }
        frame "psth" {
          n135 = control-ref of="PSTH"() -> (w236:refnum<vi>)
          n136 = call "PSTR-Show PSTHs.vi"("Data"=w235, "XYGraph"=w236, "Freq"="iFreq 2", "Separation"="Separation (uV)", "Show fits"="Show fits") -> ()  [unwired: 11 in]
        }
        frame "amplitude" {
          n137 = control-ref of="RespAmp"() -> (w239:refnum<vi>)
          n138 = local read "iFreq 2"() -> (w241:u16)
          n139 = call "PSTR-Plot Response Amplitudes.vi"("Data"=w240, "XYGraph"=w239, "Freq index"=w241) -> ()  [unwired: 13 in]
        }
        frame "reanalyze" {
          n140 = local read "Path"() -> (w249:path)
          n141 = Bundle(enum16{"Reprocess", "Export"}."Reprocess", "Path"=w249, "PSTR Params"=w248) -> (w247:T59)  [unwired: 1 in]
          n142 = Enqueue Element(queue=w246, element=w247) -> ()  [unwired: 2 in, 3 out]
        }
        frame "restore" {
          n143 = call "Default Config File Path.vi"() -> ("Default config file name"=w263:path)
          n144 = call "Read Anything.vi"("Type of Anything"=w257, "Section Name (Name of \"Type of Anything\")"="PSTRA" ("Section Name (Name of \"Type of Anything\")"), "Path (dialog)"=w263) -> ("Error Out"=w262:errorcluster, "Found?"=w259:bool, "Anything"=w261:variant)  [unwired: 6 in]
          n145 = case shown="True" w259 {
            tunnel: w262 -> [w266 w272]
            tunnel: w261 -> [_ w271]
            tunnel: [w267 w270] -> w255
            tunnel: [w266 w269] -> w260
            tunnel: w257 -> [w267 w268]
            frame False {
            }
            frame True {
              n146 = Variant To Data(error in=w272, type=w268, Variant=w271) -> (data=w270:T19, error out=w269:errorcluster)
            }
          }
          n147 = Unbundle By Name(w255) -> ("Last folder"=w254:path, "separation"=w253:dbl)
          n148 = call "Error Handler.vi"("error in (no error)"=w260) -> ()  [unwired: 13 in, 2 out]
          n149 = property on="Path" class="Path"("StartPath"=w254) -> ()  [unwired: 2 in, 2 out]
          n150 = local write "Separation (uV)"(w253) -> ()
        }
        frame "ring" {
          n151 = Unbundle By Name(w282) -> ("Freq"=w285:dbl[], "order"=w279:i32[])
          n152 = local read "iFreq 2"() -> (w273:u16)
          n153 = local read "iFreq"() -> (w281:u16)
          n154 = Array Size(array=w279) -> (size(s)=w278:i32)
          n155 = Sort 1D Array(array=w279) -> (sorted array=w284:i32[])
          n156 = for {
            tunnel: w284 -> [w292] mode=indexing
            tunnel: [w289] -> w277 mode=indexing
            tunnel: w285 -> [w291]
            n157 = Index Array(array=w291, index=w292) -> (element=w290:dbl)
            n158 = Format Into String(format string="%#_4g kHz", w290) -> (resulting string=w293:string)  [unwired: 2 in, 1 out]
            n159 = Bundle(w293, "Freq"=w292) -> (w289:cluster{string, "Freq":i32})  [unwired: 1 in]
          }
          n160 = Decrement(x=w278) -> (x-1=w275:i32)
          n161 = Max & Min(x=w275, y=w281) -> (min(x,y)=w280:i32)  [unwired: 1 out]
          n162 = Max & Min(x=w275, y=w273) -> (min(x,y)=w274:i32)  [unwired: 1 out]
          n163 = control-ref of="iFreq"() -> (w283:refnum<vi>)
          n164 = control-ref of="iFreq 2"() -> (w276:refnum<vi>)
          n165 = property class="Ring (strict)"(reference=w276, "StringsAndValues[]"=w277, "Value"=w274) -> ()  [unwired: 1 in, 2 out]
          n166 = property class="Ring (strict)"(reference=w283, "StringsAndValues[]"=w277, "Value"=w280) -> ()  [unwired: 1 in, 2 out]
        }
        frame "summary" {
          n167 = control-ref of="vsFreq"() -> (w297:refnum<vi>)
          n168 = call "PSTR-Show Summary.vi"("Data"=w296, "XYGraph"=w297) -> ()  [unwired: 14 in]
        }
      }
      n169 = Empty Array?(array=w119) -> (empty?=w125:bool)
    }
  }
  n170 = disable-structure shown="RUN_TIME_ENGINE==True, Default" {
    disable-tunnel: w1 -> [w422 _]
    frame condition #0 {
      n171 = Quit LabVIEW(quit? (T)=w422) -> ()
    }
    frame condition #1 (active) {
    }
  }
